vi "ESIII Plot.vi"() -> ()   [LabVIEW 2012]
uses:
  Labview_Spring2014/EXO200-LabView Dec.8/LabView Dec.8/SubVi's/Time Variable.vi
  Labview_Spring2014/EXO200-LabView Dec.8/LabView Dec.8/SubVi's/Time Zone Offset.vi
  Labview_Spring2014/SQL project lib.lvlib
  <vilib>/addons/database/NI_Database_API.lvlib
panel:
  in  "Tree 2":string[](tree)=["170: Buffer Volume High Pressure Limit (torr)"]
  in  "Hours":dbl=1.0
  in  "Minutes":dbl
  in  "Seconds":dbl
  in  "Days":dbl
  in  "End time":timestamp format="%<%H:%M:%S\n%Y/%m/%d>T"
  in  "Ring":u16(ring) items=["Time Interval", "Since Start Time", "Since n Hours Ago"]
  in  "Send Data to\nWindow #":i32
  out "Num. pts.":i32
  in  "Start time":timestamp format="%<%H:%M:%S\n%Y/%m/%d>T"
  in  "Grab":bool
  in  "New Static\nwindow":bool
  out "Window.vi ref. array":refnum<vi>[](array[refnum])
  out "error out":errorcluster
  out "Window counter":i32
  # "Select Data Channel"
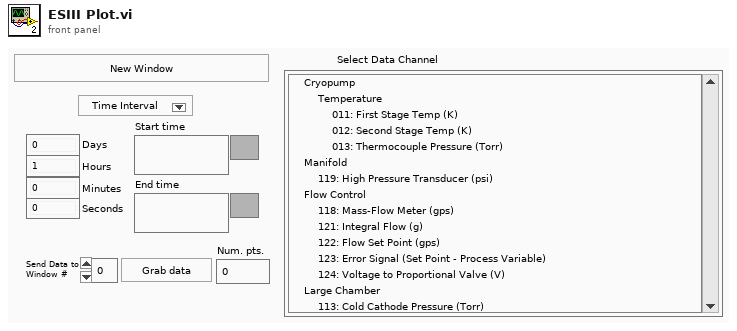
[diagram p1: front panel]
types:
  T1 = cluster{"Command":string, "Array of XY graphs":cluster{"Time":dbl[], "Y-values":dbl[]}[], "vi reference":refnum<vi>, "Data name":string, "Realtime?":bool}
  T2 = enum32{"Invalid", "Standard", "Closed", "Hidden", "Minimized", "Maximized"}
  T3 = typedef "NI_Database_API.lvlib/Conn ObjectReference.ctl" = refnum<k1>
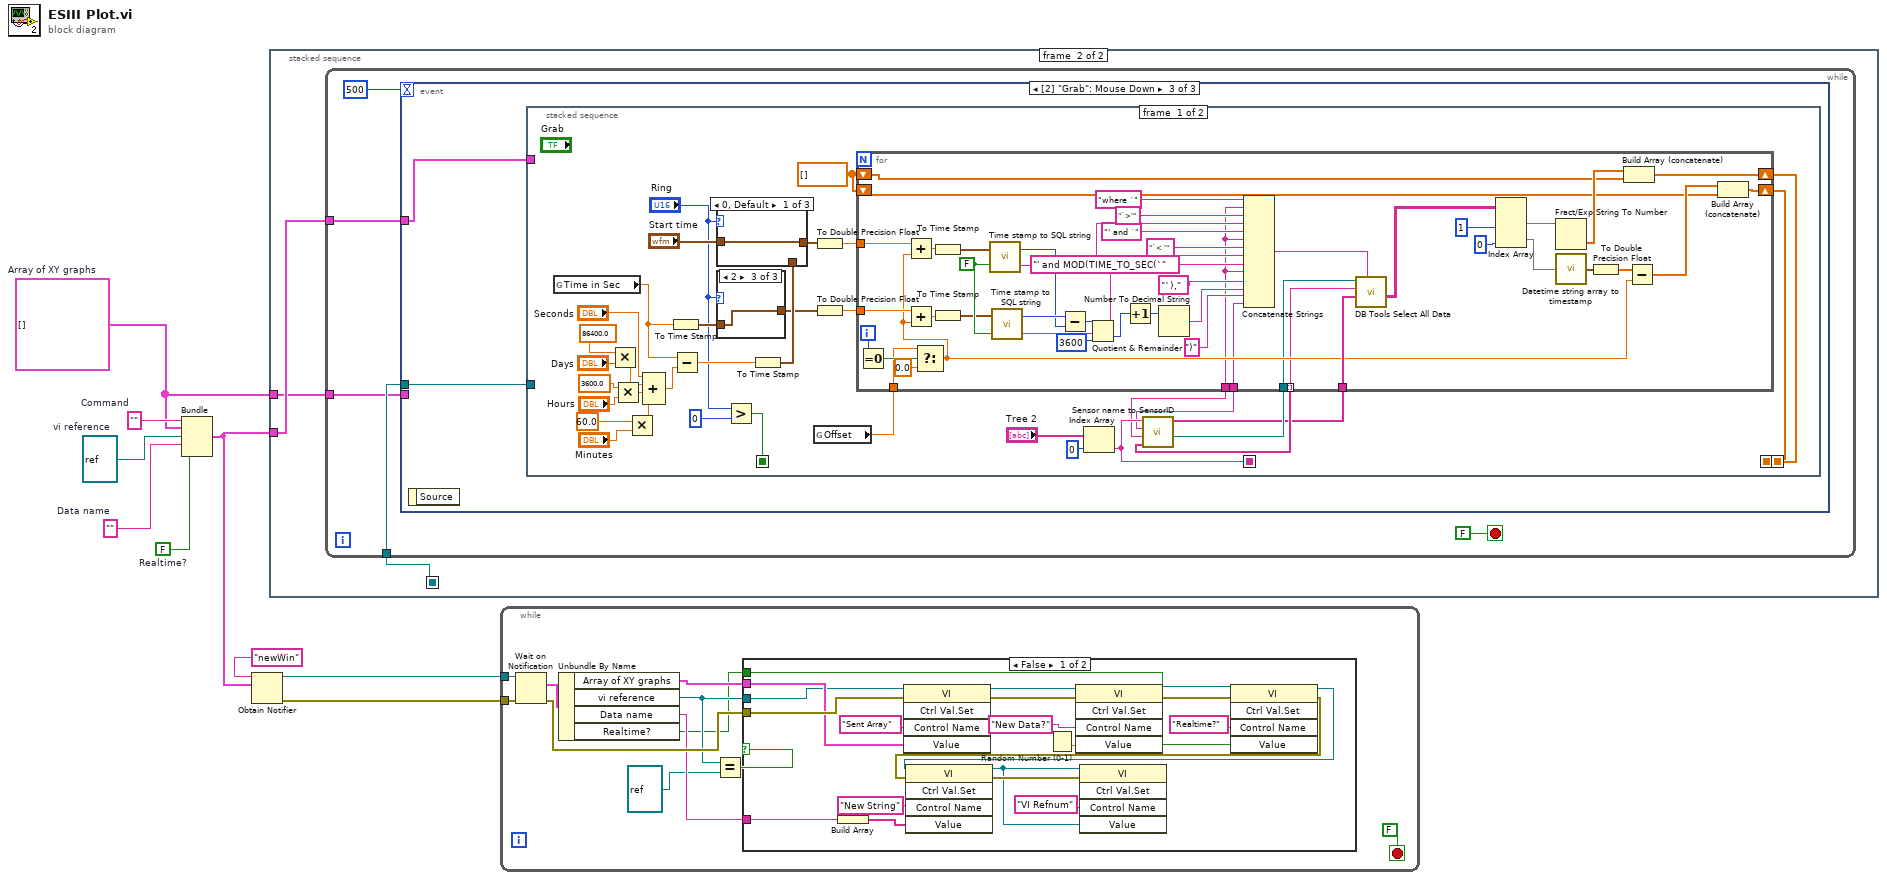
[diagram p0: block diagram]
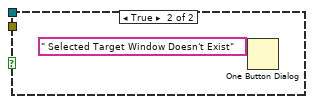
[diagram p2: hidden frame]
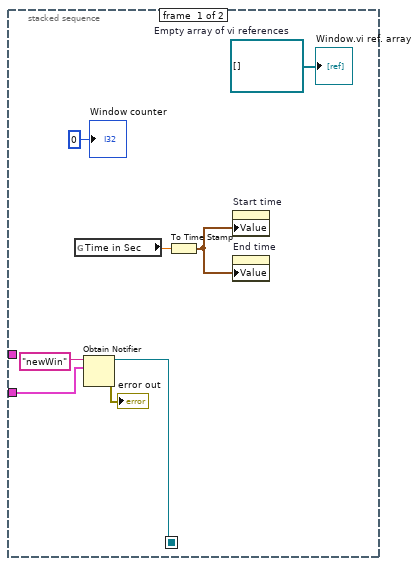
[diagram p3: hidden frame]
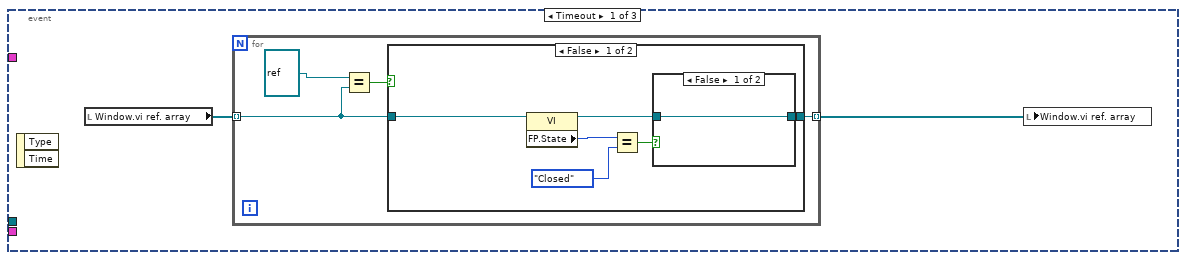
[diagram p4: hidden frame]
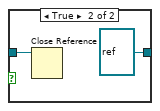
[diagram p5: hidden frame]
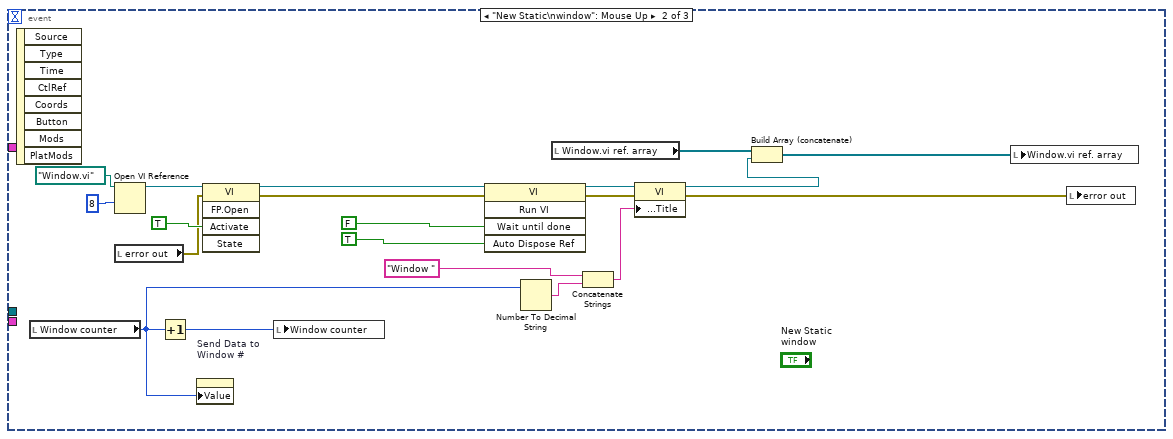
[diagram p7: hidden frame]
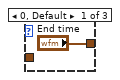
[diagram p10: hidden frame]
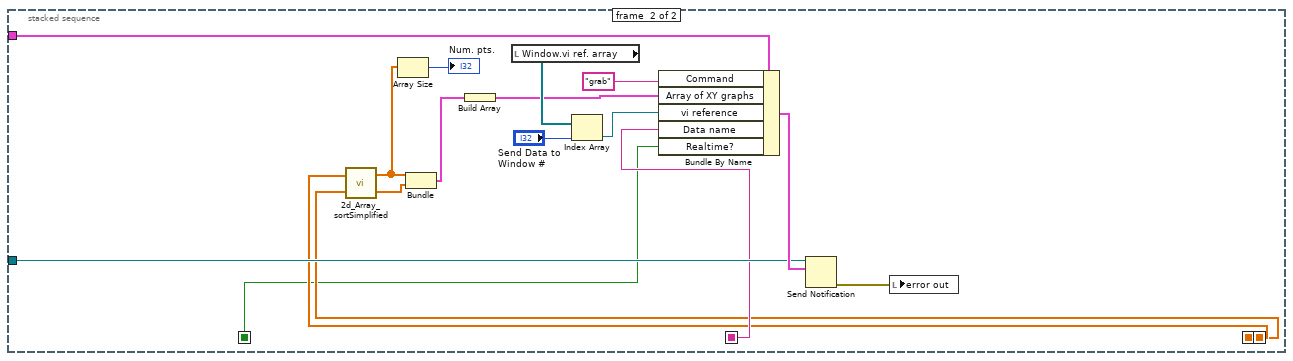
[diagram p12: hidden frame]
diagram:
  w1 = FALSE  # Realtime?
  w2 = cluster{"Time":dbl[], "Y-values":dbl[]}[] []  # Array of XY graphs
  w3 = ""  # Data name
  w8 = refnum<vi> refnum  # vi reference
  w9 = ""  # Command
  n1 = Bundle("Command"=w9, "Array of XY graphs"=w2, "vi reference"=w8, "Data name"=w3, "Realtime?"=w1) -> (w4:T1)  [unwired: 1 out]
  n2 = Obtain Notifier(name (unnamed)="newWin", notification data type=w4) -> (notifier out=w6:refnum<notifier>, error out=w5:errorcluster)  [unwired: 2 in, 1 out]
  n3 = stacked-sequence {
    seq-local: [w17 _] -> [_ w20]
    tunnel: w4 -> [w15 w19]
    tunnel: w2 -> [_ w18]
    frame #0 {
      w16 = refnum<vi>[] []  # Empty array of vi references
      n4 = global read "Time Variable.vi" "Time in Sec"() -> (w11:dbl)
      n5 = Obtain Notifier(name (unnamed)="newWin", notification data type=w15) -> (notifier out=w17:refnum<notifier>, error out=→"error out":errorcluster)  [unwired: 2 in, 1 out]
      n6 = To Time Stamp(1:w11) -> (0:w10:timestamp)
      n7 = property on="Start time" class="AbsTime (strict)"("Value"=w10) -> ()  [unwired: 2 in, 2 out]
      n8 = property on="End time" class="AbsTime (strict)"("Value"=w10) -> ()  [unwired: 2 in, 2 out]
      "Window.vi ref. array" <- w16
      "Window counter" <- 0 ("Window counter")
    }
    frame #1 {
      n9 = while {
        tunnel: w20 -> [w24]
        tunnel: w19 -> [w23]
        tunnel: w18 -> [w22]
        stop <- FALSE ("Stop VI") stop-if-true
        n10 = event shown="[2] \"Grab\": Mouse Down" {
          selector: _ -> [_ _ _]
          dyn-events: _ -> [_ _ _]
          timeout: 500 -> [_ _ _]
          tunnel: w24 -> [_ _ w62]
          tunnel: w23 -> [_ _ w63]
          tunnel: w22 -> [_ _ _]
          event Timeout {
            n11 = event-data() -> ()  [unwired: 3 out]
            n12 = local read "Window.vi ref. array"() -> (w27:refnum<vi>[])
            n13 = for {
              tunnel: w27 -> [w28] mode=indexing
              tunnel: [w31] -> w26 mode=indexing
              n14 = Equal?(x=refnum<vi> refnum, y=w28) -> (x = y?=w30:bool)
              n15 = case shown="False" w30 {
                tunnel: w28 -> [w37 w41]
                tunnel: [w32 w41] -> w31
                frame False {
                  n16 = property class="VI"(reference=w37) -> (reference out=w36:refnum<vi>, "FP.State"=w35:T2)  [unwired: 1 in, 1 out]
                  n17 = Equal?(x=w35, y=T2."Closed") -> (x = y?=w34:bool)
                  n18 = case shown="False" w34 {
                    tunnel: w36 -> [w38 w40]
                    tunnel: [w38 refnum<vi> refnum] -> w32
                    frame False {
                    }
                    frame True {
                      n19 = Close Reference(reference=w40) -> ()  [unwired: 1 in, 1 out]
                    }
                  }
                }
                frame True {
                }
              }
            }
            n20 = local write "Window.vi ref. array"(w26) -> ()
          }
          event "New Static\nwindow": Mouse Up {
            n21 = event-data() -> ()  [unwired: 9 out]
            n22 = local read "Window counter"() -> (w44:i32)
            n23 = Open VI Reference(vi path=path "Window.vi", options=8) -> (vi reference=w58:refnum<vi>)  [unwired: 1 in, 4 out]
            n24 = local read "error out"() -> (w48:errorcluster)
            n25 = Increment(x=w44) -> (x+1=w45:i32)
            n26 = property on="Send Data to\nWindow #" class="DigNum (strict)"("Value"=w44) -> ()  [unwired: 2 in, 2 out]
            n27 = invoke class="VI" method="FP.Open"(reference=w58, error in=w48, "Activate"=TRUE ("Activate?")) -> (reference out=w57:refnum<vi>, error out=w56:errorcluster)  [unwired: 2 in, 3 out]
            n28 = local write "Window counter"(w45) -> ()
            n29 = invoke class="VI" method="Run VI"(reference=w57, error in=w56, "Wait until done"=FALSE ("Wait Until Done"), "Auto Dispose Ref"=TRUE ("Auto Dispose Reference")) -> (reference out=w53:refnum<vi>, error out=w52:errorcluster)  [unwired: 1 in, 3 out]
            n30 = Number To Decimal String(number=w44) -> (decimal integer string=w51:string)  [unwired: 1 out]
            n31 = local read "Window.vi ref. array"() -> (w47:refnum<vi>[])
            n32 = Concatenate Strings("Window " ("string"), w51) -> (w49:string)
            n33 = property class="VI"(reference=w53, error in=w52, "Front Panel.Title"=w49) -> (reference out=w43:refnum<vi>, error out=w42:errorcluster)
            n34 = Build Array (concatenate)(w47, w43) -> (w46:refnum<vi>[])
            n35 = local write "Window.vi ref. array"(w46) -> ()
            n36 = local write "error out"(w42) -> ()
          }
          event "Grab": Mouse Down {
            n37 = event-data() -> ()  [unwired: 2 out]
            n38 = stacked-sequence {
              seq-local: [w77 _] -> [_ w157]
              seq-local: [w75 _] -> [_ w154]
              seq-local: [w76 _] -> [_ w153]
              seq-local: [w71 _] -> [_ w152]
              tunnel: w63 -> [_ w165]
              tunnel: w62 -> [_ w160]
              frame #0 {
                w74 = dbl[] []
                n39 = global read "Time Variable.vi" "Time in Sec"() -> (w83:dbl)
                n40 = Multiply(x=86400.0 ("disabled index (col)"), y="Days") -> (x*y=w95:dbl)
                n41 = Multiply(x=3600.0 ("disabled index (col)"), y="Hours") -> (x*y=w96:dbl)
                n42 = Multiply(x=60.0 ("disabled index (col)"), y="Minutes") -> (x*y=w97:dbl)
                n43 = Compound Arithmetic op=ADD("Seconds", w95, w96, w97) -> (w91:dbl)
                n44 = To Time Stamp(1:w83) -> (0:w82:timestamp)
                n45 = Subtract(x=w83, y=w91) -> (x-y=w85:dbl)
                n46 = case shown="2" "Ring" {
                  tunnel: ["End time" w150 w151] -> w80
                  tunnel: w82 -> [_ w150 w151]
                  frame 0, Default {
                  }
                  frame 1 {
                  }
                  frame 2 {
                  }
                }
                n47 = Greater?(x="Ring", y=u16 0) -> (0:w71:bool)
                n48 = To Time Stamp(1:w85) -> (0:w84:timestamp)
                n49 = case shown="0, Default" "Ring" {
                  tunnel: [w146 w147 w148] -> w81
                  tunnel: "Start time" -> [w146 w147 _]
                  tunnel: w84 -> [_ _ w148]
                  frame 0, Default {
                  }
                  frame 1 {
                  }
                  frame 2 {
                  }
                }
                n50 = global read "Time Zone Offset.vi" "Offset"() -> (w64:dbl)
                n51 = To Double Precision Float(number=w81) -> (double precision float=w79:dbl)
                n52 = To Double Precision Float(number=w80) -> (double precision float=w78:dbl)
                n53 = Index Array(array="Tree 2", index=0) -> (element=w77:string)
                n54 = call "Sensor name to SensorID.vi"("Sensor name"=w77) -> ("Database Connection"=w69:T3, "Column Names"=w66:string[], "TableNameArray"=w70:string[], "Time Name"=w67:string, "Modulus Number"=w68:string)  [unwired: 2 out]
                n55 = for {
                  tunnel: w66 -> [w145]
                  tunnel: w79 -> [w144]
                  tunnel: w78 -> [w143]
                  tunnel: w64 -> [w125]
                  shift-right: [w114] -> w76
                  shift-left: w74 -> [w111]
                  shift-right: [w112] -> w75
                  shift-left: w74 -> [w110]
                  tunnel: w70 -> [w109] mode=indexing
                  tunnel: w69 -> [w108]
                  tunnel: w68 -> [w100]
                  tunnel: w67 -> [w99]
                  i -> [w127]
                  w142 = FALSE ("SQL formatting?")
                  n56 = Equal To 0?(x=w127) -> (x = 0?=w126:bool)
                  n57 = Select(t=w125, s=w126, f=0.0) -> (s? t:f=w117:dbl)
                  n58 = Add(x=w144, y=w117) -> (x+y=w129:dbl)
                  n59 = Add(x=w143, y=w117) -> (x+y=w130:dbl)
                  n60 = To Time Stamp(1:w129) -> (0:w132:timestamp)
                  n61 = To Time Stamp(1:w130) -> (0:w131:timestamp)
                  n62 = call "Time stamp to SQL string.vi"("SQL formatting?"=w142, "time stamp"=w132) -> ("SQL format date-time string"=w105:string, "Seconds Since 1904"=w139:i64)
                  n63 = call "Time stamp to SQL string.vi"("SQL formatting?"=w142, "time stamp"=w131) -> ("SQL format date-time string"=w102:string, "Seconds Since 1904"=w140:i64)
                  n64 = Subtract(x=w140, y=w139) -> (x-y=w138:i64)
                  n65 = Quotient & Remainder(x=w138, y=i64 3600) -> (floor(x/y)=w136:i64)  [unwired: 1 out]
                  n66 = Increment(x=w136) -> (x+1=w135:i64)
                  n67 = Number To Decimal String(number=w135) -> (decimal integer string=w141:string)  [unwired: 1 out]
                  n68 = Concatenate Strings("where `" ("optional clause"), w99, "`>'" ("optional clause"), w105, "' and `" ("optional clause"), w99, "`< '" ("optional clause"), w102, "' and MOD(TIME_TO_SEC(`" ("optional clause"), w99, "`)," ("optional clause"), w141, ")" ("optional clause"), w100) -> (w128:string)
                  n69 = call <vilib>:"DB Tools Select All Data.vi"("optional clause"=w128, "columns"=w145, "table"=w109, "connection reference"=w108) -> ("data"=w116:string[][])  [unwired: 1 in, 3 out]
                  n70 = Index Array(array=w116, index (col) #1=1 ("disabled index (col)"), index (col) #2=0 ("index (col)")) -> (element #1=w122:string[], element #2=w120:string[])  [unwired: 2 in]
                  n71 = Fract/Exp String To Number(string=w122) -> (number=w115:dbl[])  [unwired: 4 out]
                  n72 = call "Datetime string array to timestamp.vi"("Datetime string array"=w120) -> ("Time stamp array"=w119:timestamp[])
                  n73 = To Double Precision Float(number=w119) -> (double precision float=w118:dbl[])
                  n74 = Build Array (concatenate)(w115, w111) -> (w114:dbl[])
                  n75 = Subtract(x=w118, y=w117) -> (x-y=w113:dbl[])
                  n76 = Build Array (concatenate)(w113, w110) -> (w112:dbl[])
                }
              }
              frame #1 {
                n77 = call "2d_Array_sortSimplified.vi"("Value"=w153, "Time"=w154) -> ("Dataout"=w158:dbl[], "Timeout"=w156:dbl[])
                n78 = Array Size(array=w156) -> (size(s)=→"Num. pts.":i32)
                n79 = Bundle("Timeout"=w156, "Dataout"=w158) -> (w161:cluster{"Timeout":dbl[], "Dataout":dbl[]})  [unwired: 1 out]
                n80 = Build Array(w161) -> (w162:cluster{"Timeout":dbl[], "Dataout":dbl[]}[])
                n81 = local read "Window.vi ref. array"() -> (w163:refnum<vi>[])
                n82 = Index Array(array=w163, index="Send Data to\nWindow #") -> (element=w167:refnum<vi>)
                n83 = Bundle By Name(cluster=w165, "Command"="grab", "Array of XY graphs"=w162, "vi reference"=w167, "Data name"=w157, "Realtime?"=w152) -> (w166:T1)
                n84 = Send Notification(notification=w166, notifier=w160) -> (error out=w164:errorcluster)  [unwired: 1 in, 1 out]
                n85 = local write "error out"(w164) -> ()
              }
            }
          }
        }
      }
    }
  }
  n86 = while {
    tunnel: w6 -> [w179]
    tunnel: w5 -> [w174]
    stop <- FALSE stop-if-true
    n87 = Wait on Notification(notifier=w179, error in (no error)=w174) -> (notification=w178:T1, error out=w177:errorcluster)  [unwired: 4 out]
    n88 = Unbundle By Name(w178) -> ("Array of XY graphs"=w176:cluster{"Time":dbl[], "Y-values":dbl[]}[], "vi reference"=w170:refnum<vi>, "Data name"=w173:string, "Realtime?"=w169:bool)
    n89 = Equal?(x=w170, y=refnum<vi> refnum) -> (x = y?=w172:bool)
    n90 = case shown="False" w172 {
      tunnel: w177 -> [w199 _]
      tunnel: w176 -> [w198 _]
      tunnel: w170 -> [w197 _]
      tunnel: w173 -> [w196 _]
      tunnel: w169 -> [w180 _]
      frame False {
        n91 = Build Array(w196) -> (w189:string[])
        n92 = invoke class="VI" method="Ctrl Val.Set"(reference=w197, error in=w199, "Control Name"="Sent Array", "Value"=w198) -> (reference out=w194:refnum<vi>, error out=w193:errorcluster)  [unwired: 1 in, 3 out]
        n93 = Random Number (0-1)() -> (number: 0 to 1=w192:dbl)
        n94 = invoke class="VI" method="Ctrl Val.Set"(reference=w194, error in=w193, "Control Name"="New Data?", "Value"=w192) -> (reference out=w185:refnum<vi>, error out=w184:errorcluster)  [unwired: 1 in, 3 out]
        n95 = invoke class="VI" method="Ctrl Val.Set"(reference=w185, error in=w184, "Control Name"="Realtime?", "Value"=w180) -> (reference out=w182:refnum<vi>, error out=w183:errorcluster)  [unwired: 1 in, 3 out]
        n96 = invoke class="VI" method="Ctrl Val.Set"(reference=w182, error in=w183, "Control Name"="New String", "Value"=w189) -> (reference out=w186:refnum<vi>, error out=w187:errorcluster)  [unwired: 1 in, 3 out]
        n97 = invoke class="VI" method="Ctrl Val.Set"(reference=w186, error in=w187, "Control Name"="VI Refnum", "Value"=w186) -> ()  [unwired: 1 in, 5 out]
      }
      frame True {
        n98 = One Button Dialog(message=" Selected Target Window Doesn't Exist") -> ()  [unwired: 2 out]
      }
    }
  }
